vi "Read Waveform.vi"(8 "error in (no error)":errorcluster, 10 "Channel":T1, 11 "PXIe5105 in":refnum<class "PXIe5105.lvclass">) -> (0 "error out":errorcluster, 2 "Waveform":waveform(dbl)(graph), 3 "PXIe5105 out":refnum<class "PXIe5105.lvclass">)   [LabVIEW 2018, in "PXIe5105.lvlib" / "PXIe5105.lvclass"]
doc: "This Override method is used to initiate waveform acquisition. Select targeted channel at the 'Channel' control and output waveform data to the 'Waveform' indicator."
uses:
  PXIe5105.lvclass
  PPLs/Oscilloscope/Parent/Oscilloscope.lvlibp/Custom Controls/Analog Channels.ctl
  PXIe5105.lvclass/PXIe5105.ctl
  <instrlib>/niScope/Acquire/Fetch/niScope Fetch WDT.vi
  PPLs/Oscilloscope/Parent/Oscilloscope.lvlibp
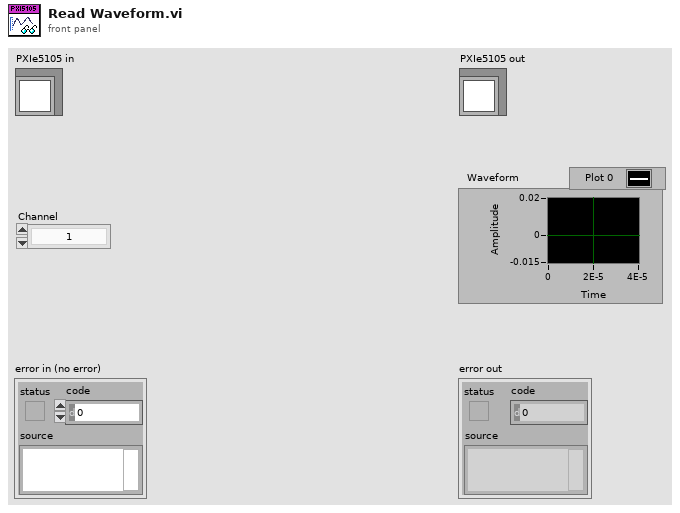
[diagram p1: front panel]
types:
  T1 = typedef "Oscilloscope.lvlibp/Analog Channels.ctl" = enum16{"1", "2", "3", "4", "5", "6", "7", "8", "9", "10", "11", "12", "13", "14", "15", "16"}
  T2 = typedef "niScope timestamp type.ctl" = i32
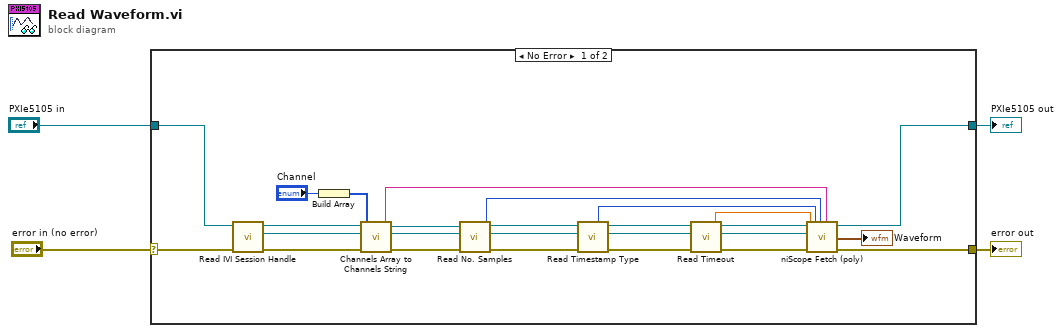
[diagram p0: block diagram]
diagram:
  n1 = case shown="No Error" "error in (no error)" {
    selector: "error in (no error)" -> [w20 w27]
    tunnel: [w6 w27] -> w3
    tunnel: [w15 w26] -> w2
    tunnel: "PXIe5105 in" -> [w21 w26]
    frame No Error {
      n2 = call "Read IVI Session Handle.vi"("error in (no error)"=w20, "PXIe5105 in"=w21) -> ("error out"=w18:errorcluster, "IVI Session Handle"=w12:refnum<k15>, "PXIe5105 out"=w19:refnum<class "PXIe5105.lvclass">)  [unwired: 7 in]
      n3 = Build Array("Channel") -> (w24:T1[])
      n4 = call "Channels Array to Channels String.vi"("error in (no error)"=w18, "Channel(s) Array"=w24, "PXIe5105 in"=w19) -> ("error out"=w23:errorcluster, "Channels String"=w11:string, "PXIe5105 out"=w22:refnum<class "PXIe5105.lvclass">)  [unwired: 6 in]
      n5 = call "Read No. Samples.vi"("error in (no error)"=w23, "PXIe5105 in"=w22) -> ("error out"=w14:errorcluster, "No. Samples"=w10:i32, "PXIe5105 out"=w17:refnum<class "PXIe5105.lvclass">)  [unwired: 7 in]
      n6 = call "Read Timestamp Type.vi"("error in (no error)"=w14, "PXIe5105 in"=w17) -> ("error out"=w13:errorcluster, "timestamp type"=w7:T2, "PXIe5105 out"=w16:refnum<class "PXIe5105.lvclass">)  [unwired: 7 in]
      n7 = call "Read Timeout.vi"("error in (no error)"=w13, "PXIe5105 in"=w16) -> ("error out"=w9:errorcluster, "Timeout"=w8:dbl, "PXIe5105 out"=w15:refnum<class "PXIe5105.lvclass">)  [unwired: 7 in]
      n8 = call-poly <instrlib>:"niScope Fetch (poly).vi"("timestamp Type"=w7, "timeout"=w8, "error in"=w9, "numSamples"=w10, "channels"=w11, "instrument handle"=w12) -> ("error out"=w6:errorcluster, "wfm"=→"Waveform":waveform(dbl))  [unwired: 2 in, 2 out]
    }
    frame Error {
    }
  }
  "error out" <- w3
  "PXIe5105 out" <- w2
